vi "waveformChartInputs.vi"() -> ()   [LabVIEW 2014]
panel:
  out "Waveform Chart\n(Multiple Waveforms, Multiple Inputs Per Iteration)":T1(graph)
  out "Waveform Chart\n(Multiple Waveforms, Single Input Per Iteration)":T2(graph)
  out "Waveform Chart\n(Single Waveform, Multiple Inputs Per Iteration)":waveform(dbl)(graph)
  in  "Stop Plotting":bool
  out "Waveform Chart\n(Single Waveform, Single Input Per Iteration)":dbl(graph)
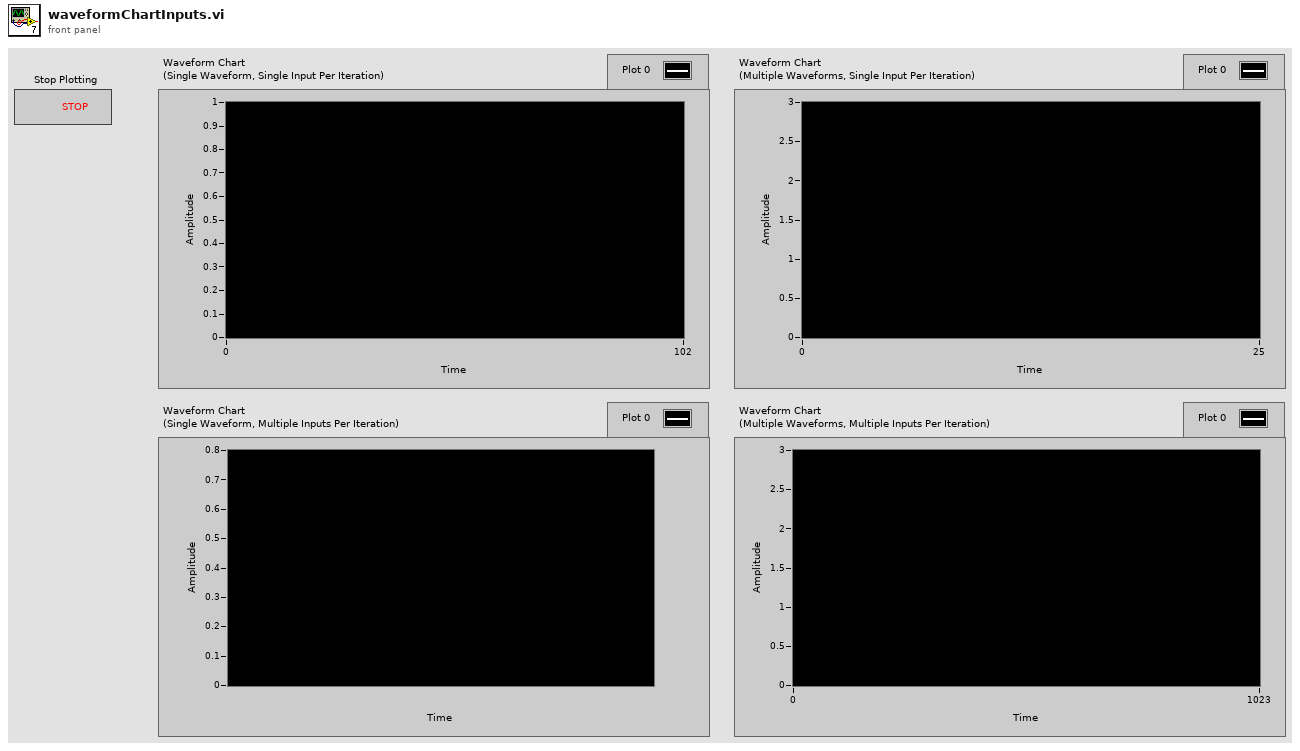
[diagram p1: front panel]
types:
  T1 = cluster{"[0]":dbl, "[1]":dbl, "[2]":dbl, "[3]":dbl, "[4]":dbl, "[5]":dbl, "[6]":dbl, "[7]":dbl, "[8]":dbl}[]
  T2 = cluster{"[0]":dbl, "[1]":dbl, "[2]":dbl, "[3]":dbl, "[4]":dbl, "[5]":dbl, "[6]":dbl, "[7]":dbl, "[8]":dbl}
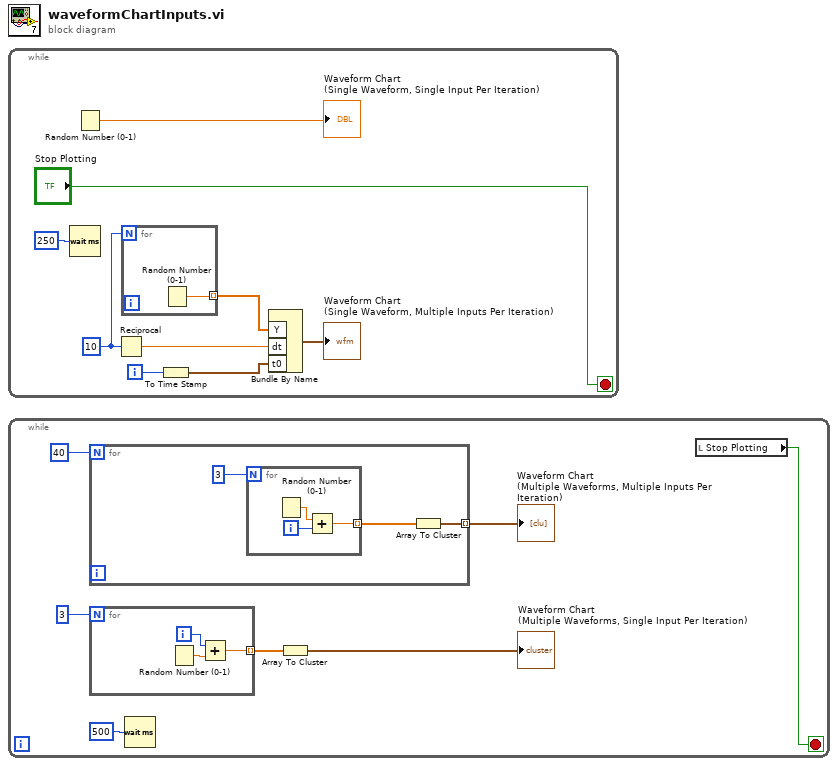
[diagram p0: block diagram]
diagram:
  n1 = while {
    i -> [w2]
    stop <- "Stop Plotting" stop-if-true
    w1 = 10
    n2 = Wait (ms)(milliseconds to wait=u32 250 ("millisecond multiple")) -> ()  [unwired: 1 out]
    n3 = Random Number (0-1)() -> (number: 0 to 1=→"Waveform Chart\n(Single Waveform, Single Input Per Iteration)":dbl)
    n4 = Reciprocal(x=w1) -> (1/x=w4:dbl)
    n5 = for {
      N: w1 -> [_]
      tunnel: [w10] -> w7 mode=indexing
      n6 = Random Number (0-1)() -> (number: 0 to 1=w10:dbl)
    }
    n7 = To Time Stamp(1:w2) -> (0:w3:timestamp)
    n8 = Bundle By Name("Y"=w7, "dt"=w4, "t0"=w3) -> (→"Waveform Chart\n(Single Waveform, Multiple Inputs Per Iteration)":waveform(dbl))  [unwired: 1 in]
  }
  n9 = while {
    stop <- w17 stop-if-true
    n10 = for {
      N: 40 -> [_]
      tunnel: [w18] -> w14 mode=indexing
      n11 = for {
        N: 3 -> [_]
        tunnel: [w23] -> w19 mode=indexing
        i -> [w21]
        n12 = Random Number (0-1)() -> (number: 0 to 1=w22:dbl)
        n13 = Add(x=w22, y=w21) -> (x+y=w23:dbl)
      }
      n14 = Array To Cluster(array=w19) -> (cluster=w18:T2)
    }
    "Waveform Chart\n(Multiple Waveforms, Multiple Inputs Per Iteration)" <- w14
    n15 = for {
      N: 3 -> [_]
      tunnel: [w24] -> w12 mode=indexing
      i -> [w25]
      n16 = Random Number (0-1)() -> (number: 0 to 1=w26:dbl)
      n17 = Add(x=w25, y=w26) -> (x+y=w24:dbl)
    }
    n18 = Wait (ms)(milliseconds to wait=u32 500 ("millisecond multiple")) -> ()  [unwired: 1 out]
    n19 = Array To Cluster(array=w12) -> (cluster=→"Waveform Chart\n(Multiple Waveforms, Single Input Per Iteration)":T2)
    n20 = local read "Stop Plotting"() -> (w17:bool)
  }
